vi "number to digits.vi"() -> ()   [LabVIEW 2020]
panel:
  out "reversed array":dbl[](array[numeric])
  in  "Numeric":dbl
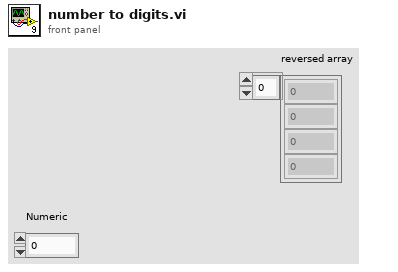
[diagram p1: front panel]
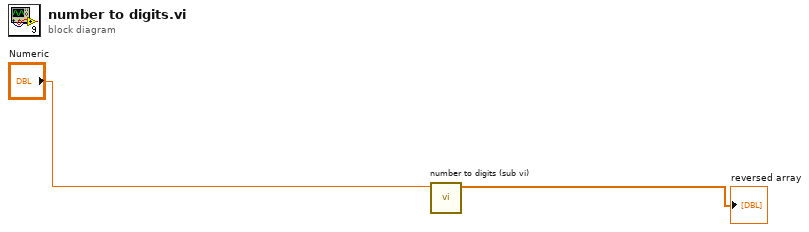
[diagram p0: block diagram]
diagram:
  n1 = call "number to digits (sub vi).vi"("Numeric"="Numeric") -> ("reversed array"=→"reversed array":dbl[])  [unwired: 10 in]
